vi "Read Measurement (Single).vi"(8 "error in (no error)":errorcluster, 9 "Timeout (10000 ms)":i32=10000, 11 "VISA resource name":refnum<visa-resource-name>) -> (0 "error out":errorcluster, 2 "Measurement":dbl, 3 "VISA resource name out":refnum<visa-resource-name>)   [LabVIEW 2019, in "Pendulum CNT90.lvlib"]
doc: "The read function performs new measurements and reads out a measuring result."
uses:
  Pendulum CNT90.lvlib
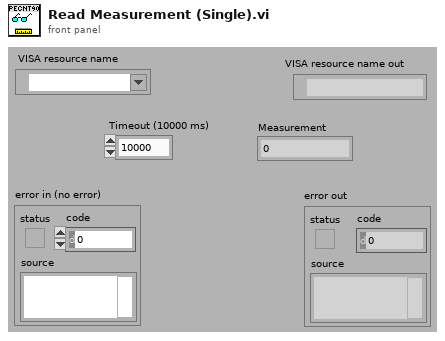
[diagram p1: front panel]
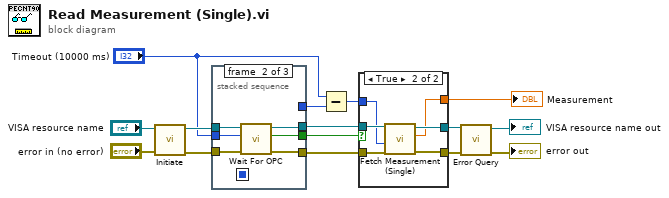
[diagram p0: block diagram]
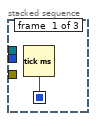
[diagram p2: hidden frame]
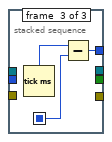
[diagram p3: hidden frame]
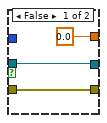
[diagram p4: hidden frame]
diagram:
  n1 = call "Initiate.vi"("error in (no error)"="error in (no error)", "VISA resource name"="VISA resource name") -> ("error out"=w4:errorcluster, "VISA resource name out"=w5:refnum<visa-resource-name>)  [unwired: 8 in]
  n2 = stacked-sequence {
    seq-local: [w16 _ _] -> [_ _ w24]
    tunnel: "Timeout (10000 ms)" -> [_ w19 _]
    tunnel: w5 -> [_ w18 _]
    tunnel: w4 -> [_ w20 _]
    tunnel: [_ w21 _] -> w14
    tunnel: [_ w22 _] -> w15
    tunnel: [_ _ w23] -> w13
    tunnel: [_ w17 _] -> w11
    frame #0 {
      n3 = Tick Count (ms)() -> (millisecond timer value=w16:u32)
    }
    frame #1 {
      n4 = call "Wait For OPC.vi"("error in (no error)"=w20, "Timeout (10000 ms)"=w19, "VISA resource name"=w18) -> ("error out"=w21:errorcluster, "Complete"=w17:bool, "VISA resource name out"=w22:refnum<visa-resource-name>)  [unwired: 6 in]
    }
    frame #2 {
      n5 = Tick Count (ms)() -> (millisecond timer value=w25:u32)
      n6 = Subtract(x=w25, y=w24) -> (x-y=w23:u32)
    }
  }
  n7 = Subtract(x="Timeout (10000 ms)", y=w13) -> (x-y=w12:u32)
  n8 = case shown="True" w11 {
    tunnel: w15 -> [w28 w34]
    tunnel: w14 -> [w27 w33]
    tunnel: [w28 w32] -> w8
    tunnel: [w27 w31] -> w7
    tunnel: w12 -> [_ w30]
    tunnel: [0.0 ("Result") w29] -> w6
    frame False {
    }
    frame True {
      n9 = call "Fetch Measurement (Single).vi"("error in (no error)"=w33, "Timeout (10000 ms)"=w30, "VISA resource name"=w34) -> ("error out"=w31:errorcluster, "Measurement"=w29:dbl, "VISA resource name out"=w32:refnum<visa-resource-name>)  [unwired: 6 in]
    }
  }
  "Measurement" <- w6
  n10 = call "Error Query.vi"("error in (no error)"=w7, "VISA resource name"=w8) -> ("error out"=→"error out":errorcluster, "VISA resource name out"=→"VISA resource name out":refnum<visa-resource-name>)  [unwired: 6 in, 2 out]
